vi "max island size.vi"(10 "Coord to check":cluster{"row index":i32, "col index":i32}, 11 "not 9s = basins":bool[][](array[boolean])=[[TRUE, TRUE, FALSE, FALSE, FALSE, TRUE, TRUE, TRUE, TRUE, TRUE], [TRUE, FALSE, TRUE, TRUE, TRUE, FALSE, TRUE, FALSE, TRUE, TRUE], [FALSE, TRUE, TRUE, TRUE, TRUE, TRUE, FALSE, TRUE, FALSE, TRUE], [TRUE, TRUE, TRUE, TRUE, TRUE, FALSE, TRUE, TRUE, TRUE, FALSE], [FALSE, TRUE, FALSE, FALSE, FALSE, TRUE, TRUE, TRUE, TRUE, TRUE]]) -> (3 "size of adjacents":i32)   [LabVIEW 2018]
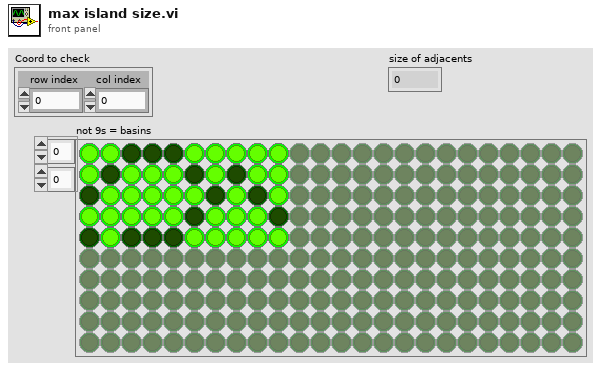
[diagram p1: front panel]
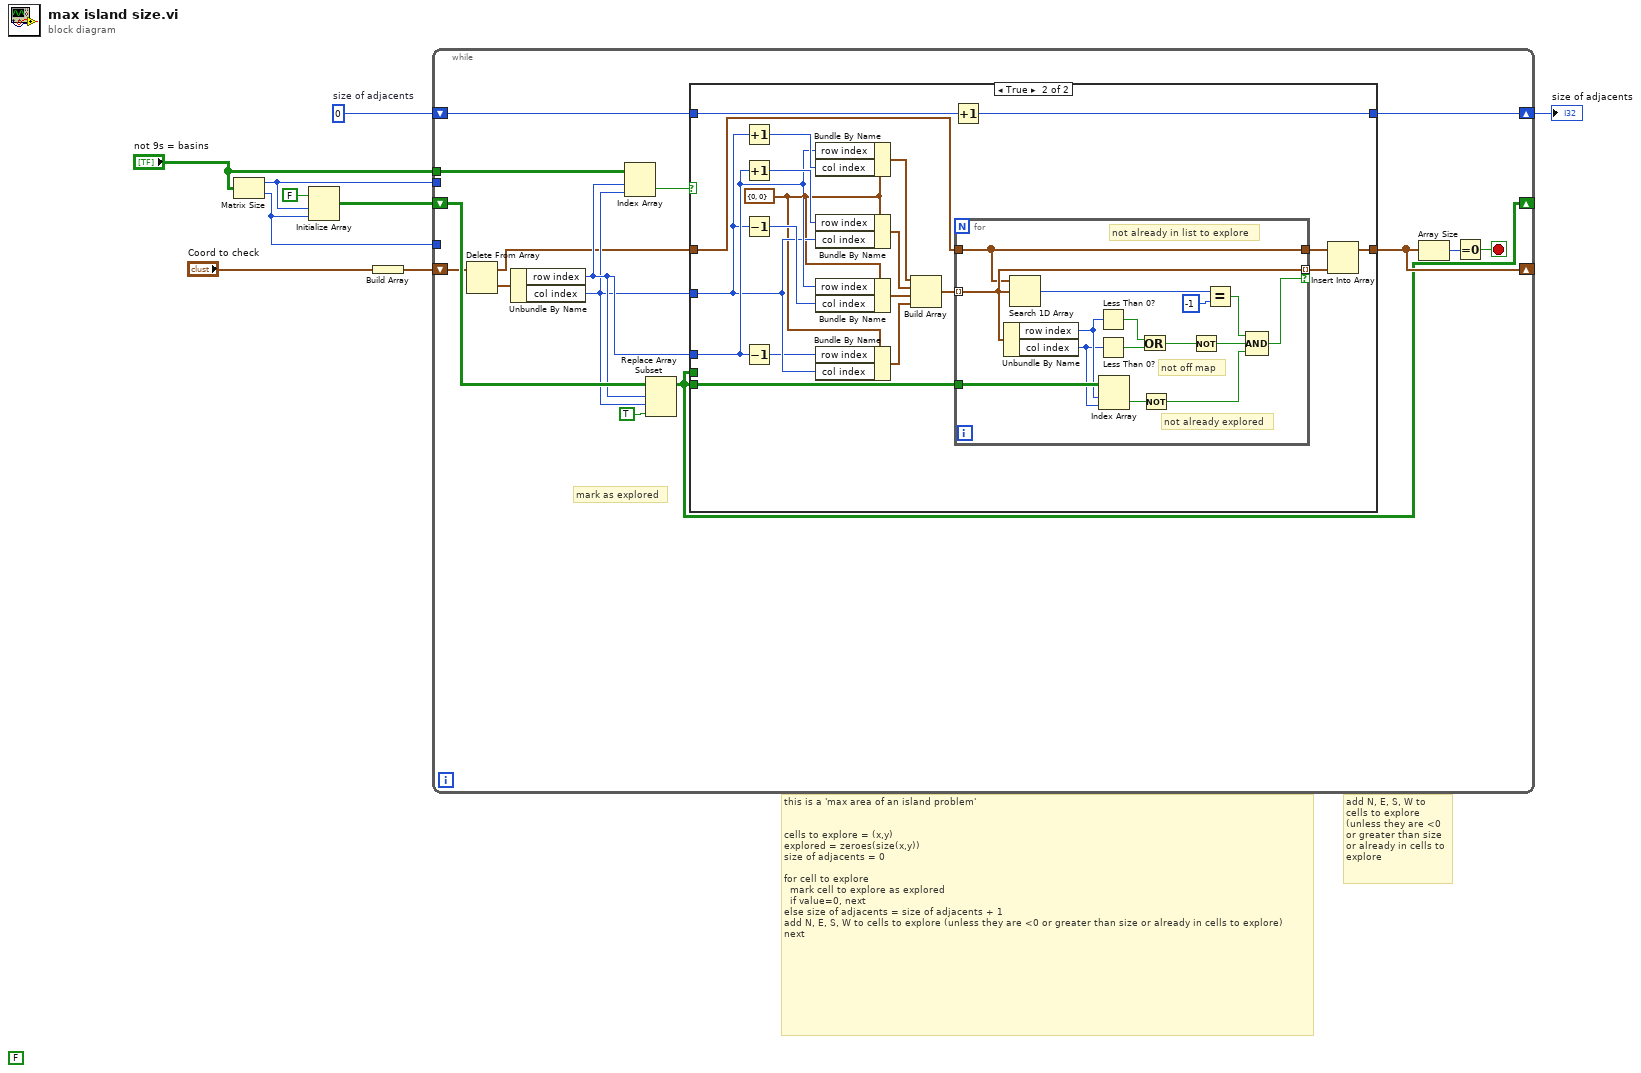
[diagram p0: block diagram]
diagram:
  w7 = 0  # size of adjacents
  (unwired) FALSE
  # "add N, E, S, W to cells to explore (unless they are <0 or greater than size or already in cells to explore"
  # "this is a 'max area of an island problem'\n\n\ncells to explore = (x,y)\nexplored = zeroes(size(x,y))\nsize of adjacents = 0\n\nfor cell to explore\n  mark cell to explore as explored\n  if value=0, next\nelse size of adjacents = size of adjacents + 1\nadd N, E, S, W to cells to explore (unless they are <0 or greater than size or already in cells to explore)\nnext"
  n1 = Matrix Size(0:"not 9s = basins") -> (1:w4:i32, 2:w3:i32)
  n2 = Initialize Array(FALSE, w4, w3) -> (w6:bool[][])
  n3 = Build Array("Coord to check") -> (w1:cluster{"row index":i32, "col index":i32}[])
  n4 = while {
    shift-right: [w20] -> w2
    shift-left: w7 -> [w21]
    shift-right: [w10] -> _
    shift-left: w6 -> [w24]
    tunnel: "not 9s = basins" -> [w17]
    tunnel: w4 -> [_]
    tunnel: w3 -> [_]
    shift-right: [w16] -> _
    shift-left: w1 -> [w12]
    stop <- w15 stop-if-true
    # "mark as explored"
    n5 = Delete From Array(array=w12) -> (deleted portion=w13:cluster{"row index":i32, "col index":i32}, array with subset deleted=w11:cluster{"row index":i32, "col index":i32}[])  [unwired: 2 in]
    n6 = Unbundle By Name(w13) -> ("row index"=w19:i32, "col index"=w18:i32)
    n7 = Index Array(array=w17, index (row)=w19, index (col)=w18) -> (element=w22:bool)
    n8 = Replace Array Subset(array=w24, new element=TRUE ("new element/subarray"), index (row)=w19, index (col)=w18) -> (w10:bool[][])
    n9 = case shown="True" w22 {
      tunnel: [w26 w44] -> w20
      tunnel: w21 -> [w26 w45]
      tunnel: w19 -> [_ w40]
      tunnel: w18 -> [_ w39]
      tunnel: w10 -> [_ _]
      tunnel: [w25 w28] -> w16
      tunnel: w11 -> [w25 w31]
      tunnel: w10 -> [_ w27]
      frame False {
        # "Move on to next"
      }
      frame True {
        w37 = cluster{"row index":i32, "col index":i32} {"row index"=0, "col index"=0}
        n10 = Increment(x=w39) -> (x+1=w43:i32)
        n11 = Increment(x=w40) -> (x+1=w42:i32)
        n12 = Decrement(x=w39) -> (x-1=w41:i32)
        n13 = Decrement(x=w40) -> (x-1=w38:i32)
        n14 = Bundle By Name(cluster=w37, "row index"=w40, "col index"=w43) -> (w36:cluster{"row index":i32, "col index":i32})
        n15 = Bundle By Name(cluster=w37, "row index"=w42, "col index"=w39) -> (w35:cluster{"row index":i32, "col index":i32})
        n16 = Bundle By Name(cluster=w37, "row index"=w40, "col index"=w41) -> (w34:cluster{"row index":i32, "col index":i32})
        n17 = Bundle By Name(cluster=w37, "row index"=w38, "col index"=w39) -> (w33:cluster{"row index":i32, "col index":i32})
        n18 = Build Array(w36, w35, w34, w33) -> (w32:cluster{"row index":i32, "col index":i32}[])
        n19 = Increment(x=w45) -> (x+1=w44:i32)
        n20 = for {
          tunnel: w32 -> [w57] mode=indexing
          tunnel: [w57] -> w29 mode=indexing if=w46
          tunnel: w31 -> [w54]
          tunnel: [w54] -> w30
          tunnel: w27 -> [w53]
          # "not already in list to explore"
          # "not off map"
          # "not already explored"
          n21 = Unbundle By Name(w57) -> ("row index"=w52:i32, "col index"=w51:i32)
          n22 = Search 1D Array(1D array=w54, element=w57) -> (index of element=w56:i32)  [unwired: 1 in]
          n23 = Less Than 0?(x=w52) -> (x < 0?=w60:bool)
          n24 = Less Than 0?(x=w51) -> (x < 0?=w59:bool)
          n25 = Index Array(array=w53, index (row)=w52, index (col)=w51) -> (element=w49:bool)
          n26 = Or(x=w60, y=w59) -> (x .or. y?=w58:bool)
          n27 = Not(x=w49) -> (.not. x?=w50:bool)
          n28 = Not(x=w58) -> (.not. x?=w48:bool)
          n29 = Equal?(x=w56, y=-1) -> (x = y?=w47:bool)
          n30 = Compound Arithmetic op=AND(w47, w48, w50) -> (w46:bool)
        }
        n31 = Insert Into Array(array=w30, new element=w29) -> (w28:cluster{"row index":i32, "col index":i32}[])  [unwired: 1 in]
      }
    }
    n32 = Array Size(array=w16) -> (size(s)=w14:i32)
    n33 = Equal To 0?(x=w14) -> (x = 0?=w15:bool)
  }
  "size of adjacents" <- w2
